vi "MGCC_FntStaMach_main_HTB.vi"() -> ()   [LabVIEW 2016]
doc: "Main function for FSM in MGCC. The inputs are flags feedback from other functions and MGLCs. The outputs are the next states and updates in sensoring datas."
panel:
  out "f_MGCC_StaEst_An":dbl[][](array[numeric])
  out "f_MGCC_StaEst_Vn":dbl[][](array[numeric])
  out "Model management":bool
  out "f_MGCC_EnergyMgmt_ISD_Ppv24":dbl[](array[numeric])
  out "f_MGCC_EnergyMgmt_Pbatt24":dbl[](array[numeric])
  out "Waveform Chart":dbl[](graph)
  in  "i_MGCC_StaEst_breakpoint":i32=11
  in  "b_MGCC_StaEst_enable_noise":bool
  out "f_MGCC_StaEst_index":dbl
  in  "b_MGCC_FntStaMach_All_Loop_Stop":bool
  out "Functions":bool[](array[boolean])
  out "Current state":string
  out "Current Time":string
  in  "Manual turn off":bool
  in  "Event manual panel":bool
  out "Bool of state":bool[](array[boolean])
  # "Finte State Machine"
  # "Energy management"
  # "State Esimation"
  # "Model Management"
  # "Data Logging"
  # "Communication"
  # "PV Forecasting"
  # "PQ Balance"
  # "Load Forecasting"
  # "BKS"
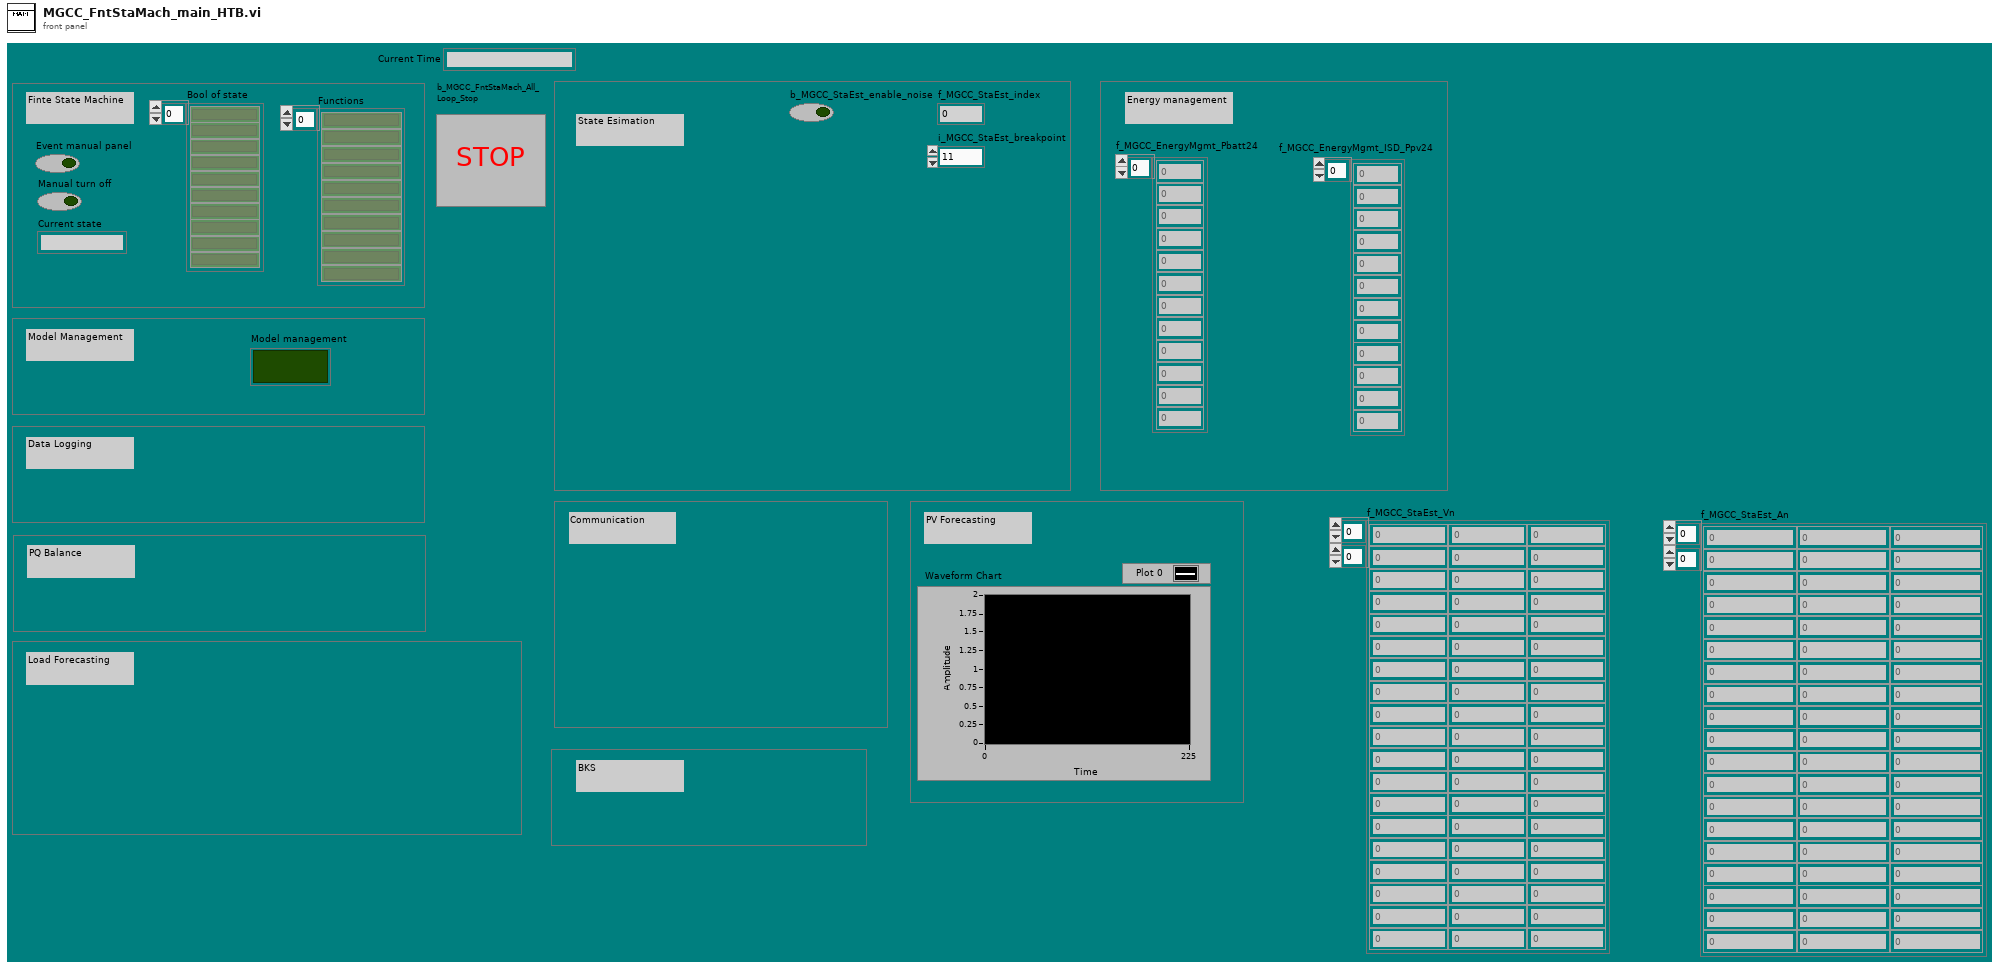
[diagram p1: front panel]
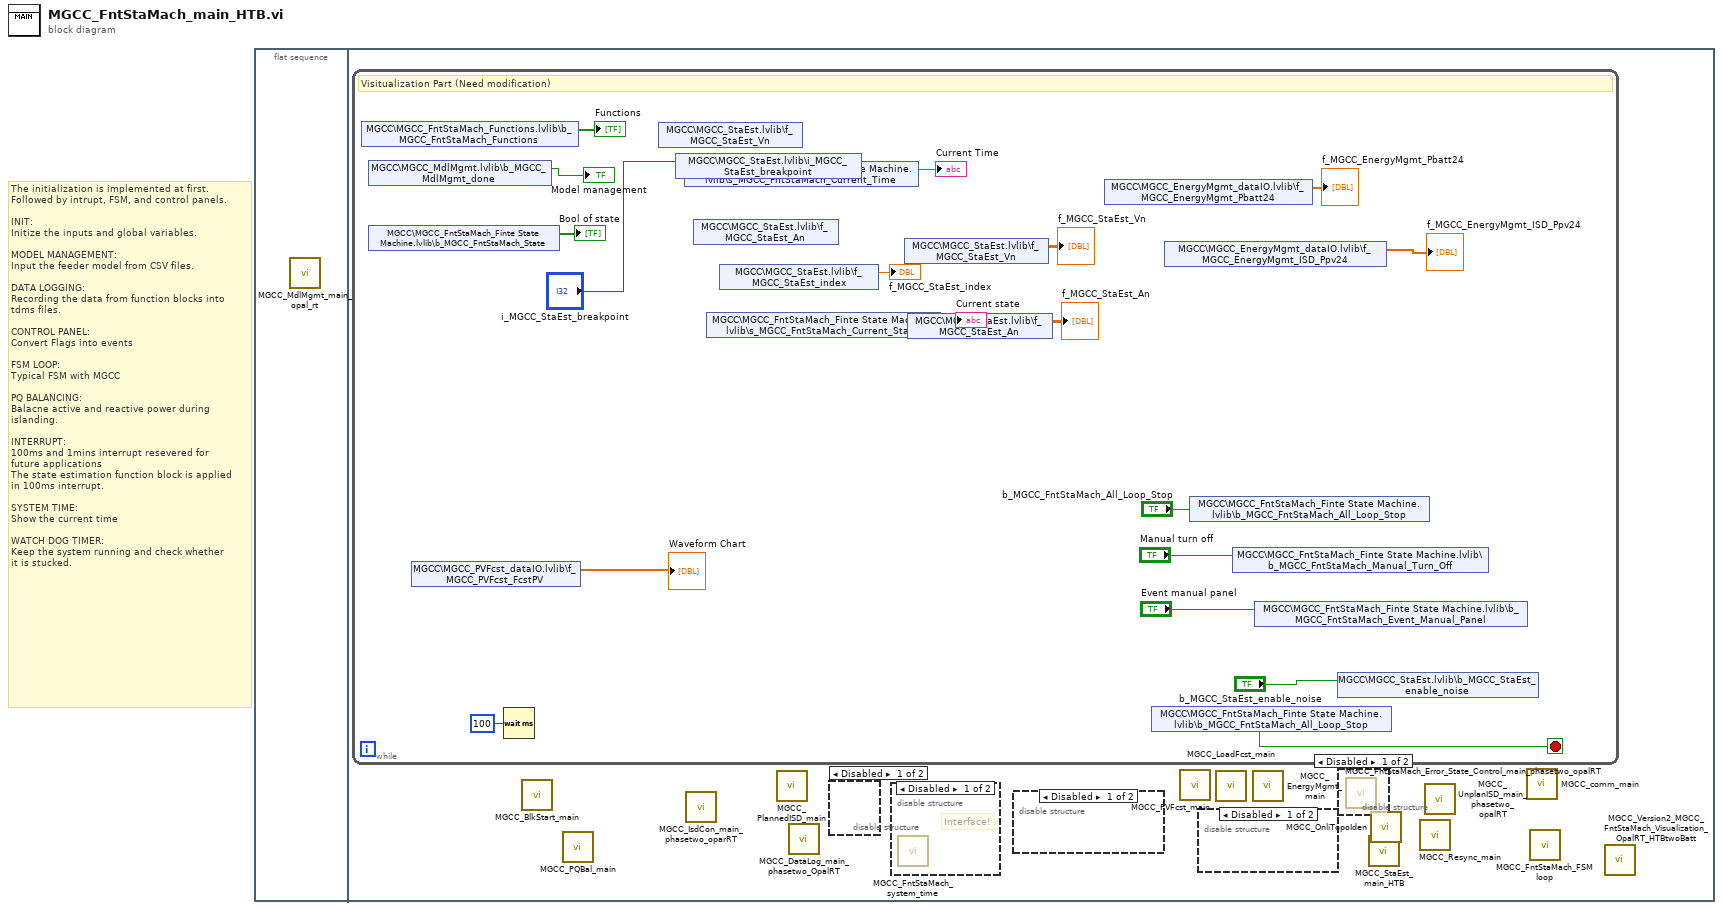
[diagram p0: block diagram]
diagram:
  # "The initialization is implemented at first.\nFollowed by intrupt, FSM, and control panels.\n\nINIT:\nInitize the inputs and global variables.\n\nMODEL MANAGEMENT:\nInput the feeder model from CSV files.\n\nDATA LOGGING:\nRecording the data from function blocks into\ntdms files.\n\nCONTROL PANEL:\nConvert Flags into events\n\nFSM LOOP:\nTypical FSM with MGCC\n\nPQ BALANCING:\nBalacne active and reactive power during \nislanding.\n\nINTERRUPT:\n100ms and 1mins interrupt resevered for \nfuture applications\nThe state estimation function block is applied\nin 100ms interrupt.\n\nSYSTEM TIME:\nShow the current time\n\nWATCH DOG TIMER:\nKeep the system running and check whether\nit is stucked."
  n1 = flat-sequence {
    frame #0 {
      n2 = call "MGCC_MdlMgmt_main_opal_rt.vi"() -> ()  [unwired: 12 in]
    }
    frame #1 {
      n3 = while {
        stop <- w17 stop-if-true
        # "Visitualization Part (Need modification)"
        n4 = shared-variable "MGCC\\MGCC_FntStaMach_Functions.lvlib\\b_MGCC_FntStaMach_Functions"() -> (→"Functions":bool[])  [unwired: 1 in, 1 out]
        n5 = shared-variable "MGCC\\MGCC_MdlMgmt.lvlib\\b_MGCC_MdlMgmt_done"() -> (→"Model management":bool)  [unwired: 1 in, 1 out]
        n6 = shared-variable "MGCC\\MGCC_FntStaMach_Finte State Machine.lvlib\\b_MGCC_FntStaMach_State"() -> (→"Bool of state":bool[])  [unwired: 1 in, 1 out]
        n7 = shared-variable "MGCC\\MGCC_PVFcst_dataIO.lvlib\\f_MGCC_PVFcst_FcstPV"() -> (→"Waveform Chart":dbl[])  [unwired: 1 in, 1 out]
        n8 = Wait (ms)(milliseconds to wait=u32 100) -> ()  [unwired: 1 out]
        n9 = shared-variable "MGCC\\MGCC_StaEst.lvlib\\f_MGCC_StaEst_Vn"() -> ()  [unwired: 1 in, 2 out]
        n10 = shared-variable "MGCC\\MGCC_StaEst.lvlib\\i_MGCC_StaEst_breakpoint"("i_MGCC_StaEst_breakpoint") -> ()  [unwired: 1 in, 1 out]
        n11 = shared-variable "MGCC\\MGCC_FntStaMach_Finte State Machine.lvlib\\s_MGCC_FntStaMach_Current_Time"() -> (→"Current Time":string)  [unwired: 1 in, 1 out]
        n12 = shared-variable "MGCC\\MGCC_StaEst.lvlib\\f_MGCC_StaEst_An"() -> ()  [unwired: 1 in, 2 out]
        n13 = shared-variable "MGCC\\MGCC_FntStaMach_Finte State Machine.lvlib\\s_MGCC_FntStaMach_Current_State"() -> (→"Current state":string)  [unwired: 1 in, 1 out]
        n14 = shared-variable "MGCC\\MGCC_StaEst.lvlib\\f_MGCC_StaEst_index"() -> (→"f_MGCC_StaEst_index":dbl)  [unwired: 1 in, 1 out]
        n15 = shared-variable "MGCC\\MGCC_StaEst.lvlib\\f_MGCC_StaEst_Vn"() -> (→"f_MGCC_StaEst_Vn":dbl[][])  [unwired: 1 in, 1 out]
        n16 = shared-variable "MGCC\\MGCC_StaEst.lvlib\\f_MGCC_StaEst_An"() -> (→"f_MGCC_StaEst_An":dbl[][])  [unwired: 1 in, 1 out]
        n17 = shared-variable "MGCC\\MGCC_EnergyMgmt_dataIO.lvlib\\f_MGCC_EnergyMgmt_Pbatt24"() -> (→"f_MGCC_EnergyMgmt_Pbatt24":dbl[])  [unwired: 1 in, 1 out]
        n18 = shared-variable "MGCC\\MGCC_FntStaMach_Finte State Machine.lvlib\\b_MGCC_FntStaMach_All_Loop_Stop"() -> (w17:bool)  [unwired: 1 in, 1 out]
        n19 = shared-variable "MGCC\\MGCC_EnergyMgmt_dataIO.lvlib\\f_MGCC_EnergyMgmt_ISD_Ppv24"() -> (→"f_MGCC_EnergyMgmt_ISD_Ppv24":dbl[])  [unwired: 1 in, 1 out]
        n20 = shared-variable "MGCC\\MGCC_FntStaMach_Finte State Machine.lvlib\\b_MGCC_FntStaMach_All_Loop_Stop"("b_MGCC_FntStaMach_All_Loop_Stop") -> ()  [unwired: 1 in, 1 out]
        n21 = shared-variable "MGCC\\MGCC_FntStaMach_Finte State Machine.lvlib\\b_MGCC_FntStaMach_Manual_Turn_Off"("Manual turn off") -> ()  [unwired: 1 in, 1 out]
        n22 = shared-variable "MGCC\\MGCC_FntStaMach_Finte State Machine.lvlib\\b_MGCC_FntStaMach_Event_Manual_Panel"("Event manual panel") -> ()  [unwired: 1 in, 1 out]
        n23 = shared-variable "MGCC\\MGCC_StaEst.lvlib\\b_MGCC_StaEst_enable_noise"("b_MGCC_StaEst_enable_noise") -> ()  [unwired: 1 in, 1 out]
      }
      n24 = call "MGCC_BlkStart_main.vi"() -> ()  [unwired: 12 in]
      n25 = call "MGCC_PQBal_main.vi"() -> ()  [unwired: 12 in]
      n26 = call "MGCC_IsdCon_main_phasetwo_oparRT.vi"() -> ()  [unwired: 12 in]
      n27 = call "MGCC_PlannedISD_main.vi"() -> ()  [unwired: 12 in]
      n28 = call "MGCC_DataLog_main_phasetwo_OpalRT.vi"() -> ()  [unwired: 12 in]
      n29 = disable-structure shown="Disabled" {
        frame Disabled {
        }
        frame Enabled {
        }
      }
      n30 = disable-structure shown="Disabled" {
        frame Disabled {
          # "Interface!"
          n31 = call "MGCC_FntStaMach_system_time.vi"() -> ()  [unwired: 12 in]
        }
        frame Enabled {
        }
      }
      n32 = disable-structure shown="Disabled" {
        frame Disabled {
        }
        frame Enabled {
        }
      }
      n33 = call "MGCC_PVFcst_main.vi"() -> ()  [unwired: 12 in]
      n34 = disable-structure shown="Disabled" {
        frame Disabled {
        }
        frame Enabled {
        }
      }
      n35 = call "MGCC_LoadFcst_main.vi"() -> ()  [unwired: 12 in]
      n36 = call "MGCC_EnergyMgmt_main.vi"() -> ()  [unwired: 12 in]
      n37 = disable-structure shown="Disabled" {
        frame Disabled {
          n38 = call "MGCC_FntStaMach_Error_State_Control_main_phasetwo_opalRT.vi"() -> ()  [unwired: 12 in]
        }
        frame Enabled {
        }
      }
      n39 = call "MGCC_StaEst_main_HTB.vi"() -> ()  [unwired: 12 in]
      n40 = call "MGCC_OnliTopoIden.vi"() -> ()  [unwired: 12 in]
      n41 = call "MGCC_Resync_main.vi"() -> ()  [unwired: 12 in]
      n42 = call "MGCC_UnplanISD_main_phasetwo_opalRT.vi"() -> ()  [unwired: 12 in]
      n43 = call "MGCC_comm_main.vi"() -> ()  [unwired: 12 in]
      n44 = call "MGCC_FntStaMach_FSM loop.vi"() -> ()  [unwired: 8 in, 4 out]
      n45 = call "MGCC_Version2_MGCC_FntStaMach_Visualization_OpalRT_HTBtwoBatt.vi"() -> ()  [unwired: 12 in]
    }
  }
